vi "subpanel.vi"(8 "error in (no error)":errorcluster, 11 "JSON string":string) -> (0 "error out":errorcluster, 3 "value":string)   [LabVIEW 2020, in "ui-testing.lvlib"]
doc: "copyright: Thomas Zilliox©"
uses:
  ui-testing.lvlib
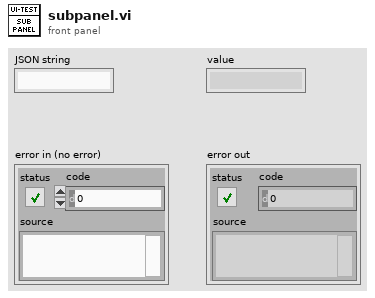
[diagram p1: front panel]
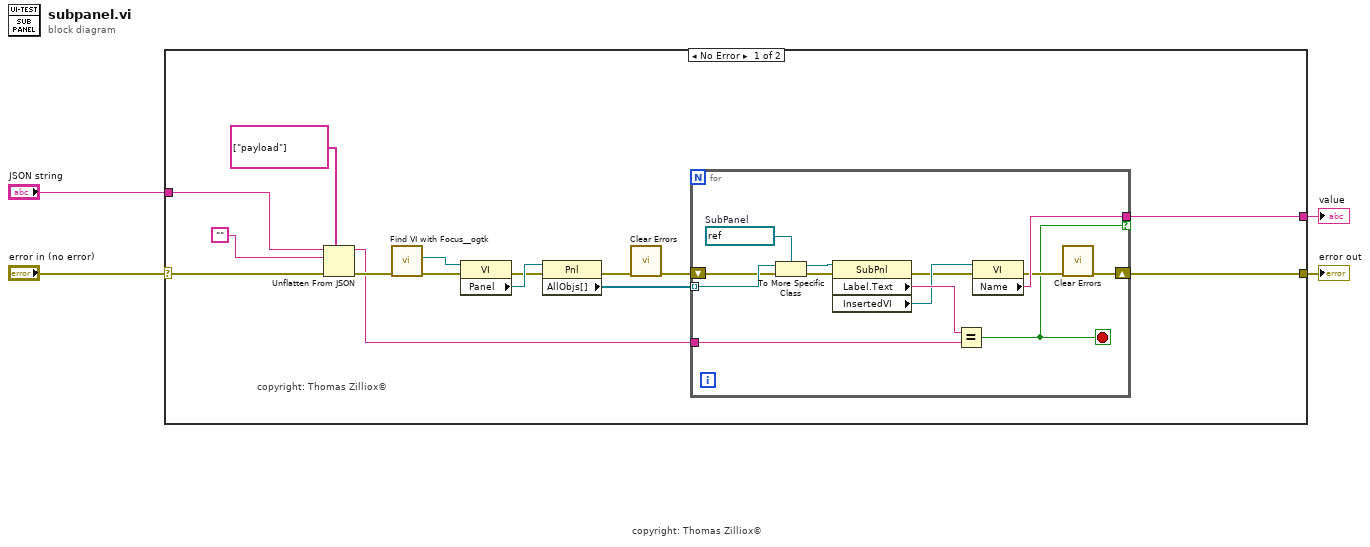
[diagram p0: block diagram]
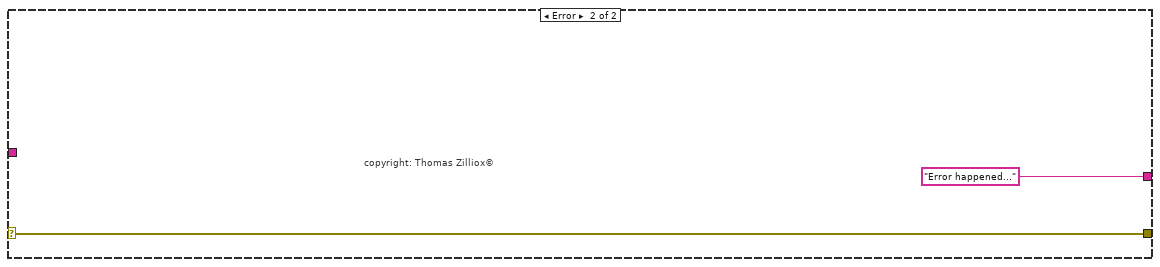
[diagram p2: hidden frame]
diagram:
  # "copyright: Thomas Zilliox©"
  n1 = case shown="No Error" "error in (no error)" {
    selector: "error in (no error)" -> [w10 w34]
    tunnel: "JSON string" -> [w12 _]
    tunnel: [w6 w34] -> w3
    tunnel: [w5 "Error happened..."] -> w1
    frame No Error {
      # "copyright: Thomas Zilliox©"
      n2 = Unflatten From JSON(path=string[] ["payload"], JSON string=w12, type and defaults="", error in (no error)=w10) -> (value=w7:string, error out=w14:errorcluster)  [unwired: 3 in]
      n3 = call <userlib>:"Find VI with Focus__ogtk.vi"("error in"=w14) -> ("error out"=w18:errorcluster, "VI with Focus"=w17:refnum<vi>)  [unwired: 6 in, 3 out]
      n4 = property class="VI"(reference=w17, error in=w18) -> (error out=w15:errorcluster, "Panel"=w16:refnum<vi>)  [unwired: 1 out]
      n5 = property class="Pnl"(reference=w16, error in=w15) -> (error out=w11:errorcluster, "AllObjs[]"=w8:refnum<vi>[])  [unwired: 1 out]
      n6 = call <vilib>:"Clear Errors.vi"("error in (no error)"=w11) -> ("error out"=w9:errorcluster)  [unwired: 5 in, 1 out]
      n7 = for {
        tunnel: w8 -> [w32] mode=indexing
        tunnel: [w26] -> w5 if=w23
        shift-right: [w20] -> w6
        shift-left: w9 -> [w22]
        tunnel: w7 -> [w21]
        stop <- w23 stop-if-true
        w31 = refnum<vi> refnum  # SubPanel
        n8 = To More Specific Class(target class=w31, reference=w32, error in=w22) -> (specific class reference=w30:refnum<vi>, error out=w29:errorcluster)
        n9 = property class="SubPnl"(reference=w30, error in=w29) -> (error out=w24:errorcluster, "Label.Text"=w28:string, "InsertedVI"=w27:refnum<vi>)  [unwired: 1 out]
        n10 = Equal?(x=w28, y=w21) -> (x = y?=w23:bool)
        n11 = property class="VI"(reference=w27, error in=w24) -> (error out=w25:errorcluster, "Name"=w26:string)  [unwired: 1 out]
        n12 = call <vilib>:"Clear Errors.vi"("error in (no error)"=w25) -> ("error out"=w20:errorcluster)  [unwired: 5 in, 1 out]
      }
    }
    frame Error {
      # "copyright: Thomas Zilliox©"
    }
  }
  "error out" <- w3
  "value" <- w1
